vi "Attributes_DAQwfm.vi"(2 "data":waveform(dbl)[](array[waveform]), 3 "Refnum in":refnum<k21>) -> (0 "Array":waveform(dbl)[](array[waveform]), 1 "Refnum in 2":refnum<k21>)   [LabVIEW 2017]
uses:
  <resource>/objmgr/daqmx.rc
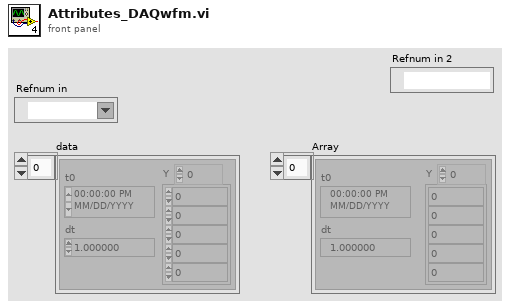
[diagram p1: front panel]
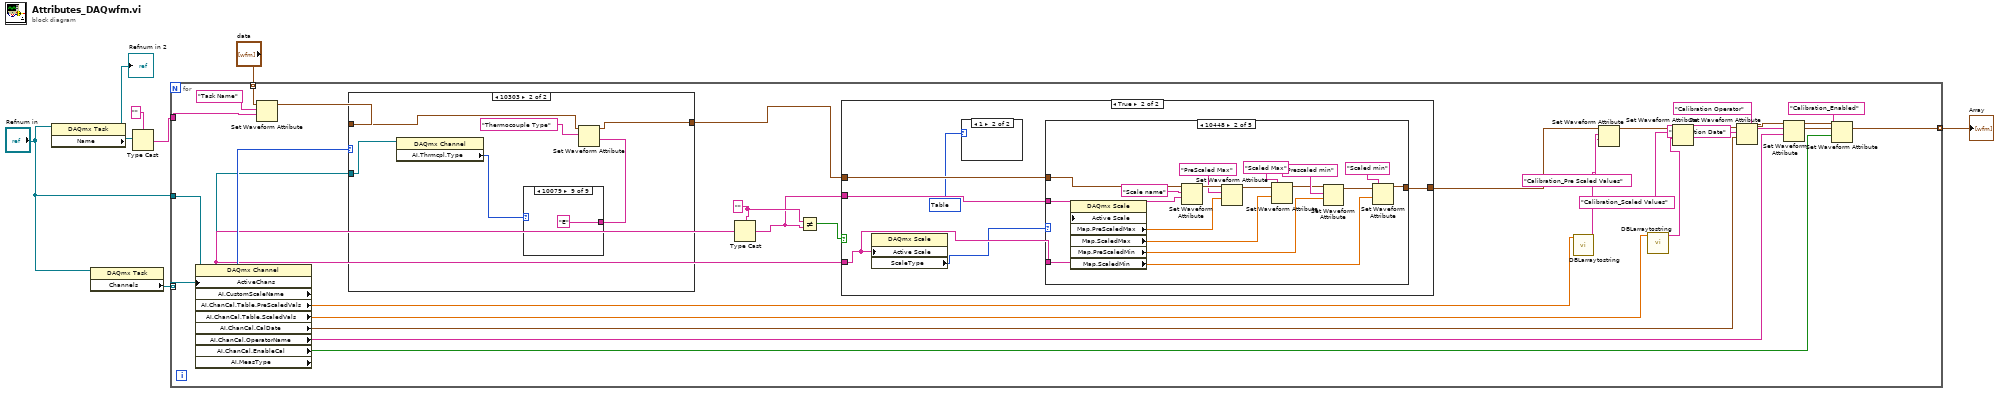
[diagram p0: block diagram]
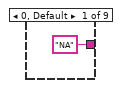
[diagram p3: hidden frame]
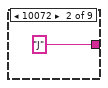
[diagram p4: hidden frame]
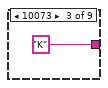
[diagram p5: hidden frame]
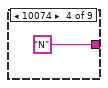
[diagram p6: hidden frame]
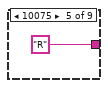
[diagram p7: hidden frame]
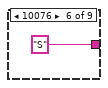
[diagram p8: hidden frame]
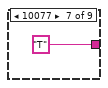
[diagram p9: hidden frame]
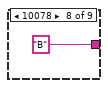
[diagram p10: hidden frame]
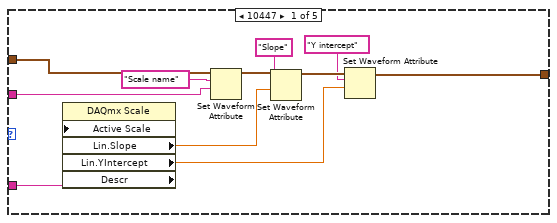
[diagram p13: hidden frame]
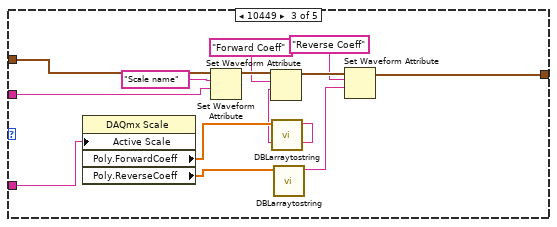
[diagram p14: hidden frame]
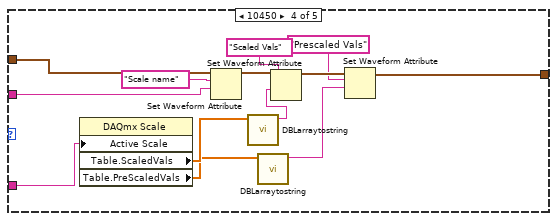
[diagram p15: hidden frame]
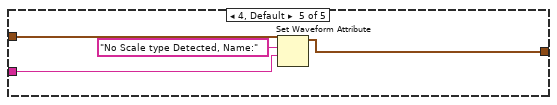
[diagram p16: hidden frame]
diagram:
  n1 = property class="DAQmx Task"(reference="Refnum in") -> (reference out=→"Refnum in 2":refnum<k21>, "Name"=w5:refnum<k21>)  [unwired: 1 in, 1 out]
  n2 = property class="DAQmx Task"(reference="Refnum in") -> ("Channels"=w2:refnum<k21>[])  [unwired: 1 in, 2 out]
  n3 = Type Cast(type="", x=w5) -> (*(type *) &x=w7:string)
  n4 = for {
    tunnel: "data" -> [w38] mode=indexing
    tunnel: [w19] -> w8 mode=indexing
    tunnel: w7 -> [w37]
    tunnel: "Refnum in" -> [w36]
    tunnel: w2 -> [w35] mode=indexing
    w18 = "" ("type")
    n5 = property class="DAQmx Channel"(reference=w36, "ActiveChans"=w35) -> (reference out=w12:refnum<k21>, "AI.CustomScaleName"=w13:tag, "AI.ChanCal.Table.PreScaledVals"=w30:dbl[], "AI.ChanCal.Table.ScaledVals"=w9:dbl[], "AI.ChanCal.CalDate"=w27:timestamp, "AI.ChanCal.OperatorName"=w25:string, "AI.ChanCal.EnableCal"=w23:bool, "AI.MeasType"=w14:i32)  [unwired: 1 in, 1 out]
    n6 = Set Waveform Attribute(5:w37, 6:"Task Name" ("name"), 7:w38) -> (3:w11:waveform(dbl))  [unwired: 1 in, 2 out]
    n7 = case shown="10303" w14 {
      tunnel: w12 -> [_ w46]
      tunnel: w11 -> [w40 w44]
      tunnel: [w40 w43] -> w10
      frame 0, Default {
      }
      frame 10303 {
        n8 = property class="DAQmx Channel"(reference=w46) -> ("AI.Thrmcpl.Type"=w42:i32)  [unwired: 1 in, 2 out]
        n9 = case shown="10079" w42 {
          tunnel: ["NA" "J" "K" "N" "R" "S" "T" "B" "E"] -> w41
          frame 0, Default {
          }
          frame 10072 {
          }
          frame 10073 {
          }
          frame 10074 {
          }
          frame 10075 {
          }
          frame 10076 {
          }
          frame 10077 {
          }
          frame 10078 {
          }
          frame 10079 {
          }
        }
        n10 = Set Waveform Attribute(5:w41, 6:"Thermocouple Type" ("name"), 7:w44) -> (3:w43:waveform(dbl))  [unwired: 1 in, 2 out]
      }
    }
    n11 = Type Cast(type=w18, x=w13) -> (*(type *) &x=w16:string)
    n12 = Not Equal?(x=w18, y=w16) -> (x != y?=w17:bool)
    n13 = case shown="True" w17 {
      tunnel: w10 -> [w56 w62]
      tunnel: [w56 w61] -> w31
      tunnel: w13 -> [_ w60]
      tunnel: w16 -> [_ w59]
      frame False {
      }
      frame True {
        w58 = 10450 items=["Linear"=10447, "Map Ranges"=10448, "Polynomial"=10449, "Table"=10450] ("ScaleType")
        n14 = property class="DAQmx Scale"("Active Scale"=w60) -> ("ScaleType"=w57:i32)  [unwired: 2 in, 2 out]
        n15 = case shown="1" w58 {
          frame 0, Default {
          }
          frame 1 {
          }
        }
        n16 = case shown="10448" w57 {
          tunnel: w62 -> [w73 w90 w103 w116 w120]
          tunnel: [w72 w76 w102 w115 w119] -> w61
          tunnel: w60 -> [w64 w82 w96 w109 _]
          tunnel: w59 -> [w63 w81 w95 w108 w117]
          frame 10447 {
            n17 = property class="DAQmx Scale" props=["Active Scale", "Lin.Slope", "Lin.YIntercept", "Descr"]("Active Scale"=w64) -> ("Lin.Slope"=w68:dbl, "Lin.YIntercept"=w67:dbl)  [unwired: 2 in, 3 out]
            n18 = Set Waveform Attribute(5:w63, 6:"Scale name" ("name"), 7:w73) -> (3:w70:waveform(dbl))  [unwired: 1 in, 2 out]
            n19 = Set Waveform Attribute(5:w68, 6:"Slope" ("name"), 7:w70) -> (3:w69:waveform(dbl))  [unwired: 1 in, 2 out]
            n20 = Set Waveform Attribute(5:w67, 6:"Y intercept" ("name"), 7:w69) -> (3:w72:waveform(dbl))  [unwired: 1 in, 2 out]
          }
          frame 10448 {
            n21 = property class="DAQmx Scale"("Active Scale"=w82) -> ("Map.PreScaledMax"=w86:dbl, "Map.ScaledMax"=w85:dbl, "Map.PreScaledMin"=w75:dbl, "Map.ScaledMin"=w74:dbl)  [unwired: 2 in, 2 out]
            n22 = Set Waveform Attribute(5:w81, 6:"Scale name" ("name"), 7:w90) -> (3:w88:waveform(dbl))  [unwired: 1 in, 2 out]
            n23 = Set Waveform Attribute(5:w86, 6:"PreScaled Max" ("name"), 7:w88) -> (3:w87:waveform(dbl))  [unwired: 1 in, 2 out]
            n24 = Set Waveform Attribute(5:w85, 6:"Scaled Max" ("name"), 7:w87) -> (3:w77:waveform(dbl))  [unwired: 1 in, 2 out]
            n25 = Set Waveform Attribute(5:w75, 6:"Prescaled min" ("name"), 7:w77) -> (3:w78:waveform(dbl))  [unwired: 1 in, 2 out]
            n26 = Set Waveform Attribute(5:w74, 6:"Scaled min" ("name"), 7:w78) -> (3:w76:waveform(dbl))  [unwired: 1 in, 2 out]
          }
          frame 10449 {
            n27 = property class="DAQmx Scale"("Active Scale"=w96) -> ("Poly.ForwardCoeff"=w94:dbl[], "Poly.ReverseCoeff"=w92:dbl[])  [unwired: 2 in, 2 out]
            n28 = Set Waveform Attribute(5:w95, 6:"Scale name" ("name"), 7:w103) -> (3:w100:waveform(dbl))  [unwired: 1 in, 2 out]
            n29 = call "DBLarraytostring.vi"("AI.ChanCal.Table.PreScaledVals"=w94) -> ("String"=w93:string)  [unwired: 10 in]
            n30 = Set Waveform Attribute(5:w93, 6:"Forward Coeff" ("name"), 7:w100) -> (3:w99:waveform(dbl))  [unwired: 1 in, 2 out]
            n31 = call "DBLarraytostring.vi"("AI.ChanCal.Table.PreScaledVals"=w92) -> ("String"=w91:string)  [unwired: 10 in]
            n32 = Set Waveform Attribute(5:w91, 6:"Reverse Coeff" ("name"), 7:w99) -> (3:w102:waveform(dbl))  [unwired: 1 in, 2 out]
          }
          frame 10450 {
            n33 = property class="DAQmx Scale"("Active Scale"=w109) -> ("Table.ScaledVals"=w107:dbl[], "Table.PreScaledVals"=w105:dbl[])  [unwired: 2 in, 2 out]
            n34 = Set Waveform Attribute(5:w108, 6:"Scale name" ("name"), 7:w116) -> (3:w113:waveform(dbl))  [unwired: 1 in, 2 out]
            n35 = call "DBLarraytostring.vi"("AI.ChanCal.Table.PreScaledVals"=w107) -> ("String"=w106:string)  [unwired: 10 in]
            n36 = call "DBLarraytostring.vi"("AI.ChanCal.Table.PreScaledVals"=w105) -> ("String"=w104:string)  [unwired: 10 in]
            n37 = Set Waveform Attribute(5:w106, 6:"Scaled Vals" ("name"), 7:w113) -> (3:w112:waveform(dbl))  [unwired: 1 in, 2 out]
            n38 = Set Waveform Attribute(5:w104, 6:"Prescaled Vals" ("name"), 7:w112) -> (3:w115:waveform(dbl))  [unwired: 1 in, 2 out]
          }
          frame 4, Default {
            n39 = Set Waveform Attribute(5:w117, 6:"No Scale type Detected, Name:" ("name"), 7:w120) -> (3:w119:waveform(dbl))  [unwired: 1 in, 2 out]
          }
        }
      }
    }
    n40 = call "DBLarraytostring.vi"("AI.ChanCal.Table.PreScaledVals"=w30) -> ("String"=w29:string)  [unwired: 10 in]
    n41 = Set Waveform Attribute(5:w29, 6:"Calibration_Pre Scaled Values" ("name"), 7:w31) -> (3:w34:waveform(dbl))  [unwired: 1 in, 2 out]
    n42 = call "DBLarraytostring.vi"("AI.ChanCal.Table.PreScaledVals"=w9) -> ("String"=w15:string)  [unwired: 10 in]
    n43 = Set Waveform Attribute(5:w15, 6:"Calibration_Scaled Values" ("name"), 7:w34) -> (3:w28:waveform(dbl))  [unwired: 1 in, 2 out]
    n44 = Set Waveform Attribute(5:w27, 6:"Calibration Date" ("name"), 7:w28) -> (3:w21:waveform(dbl))  [unwired: 1 in, 2 out]
    n45 = Set Waveform Attribute(5:w25, 6:"Calibration Operator" ("name"), 7:w21) -> (3:w20:waveform(dbl))  [unwired: 1 in, 2 out]
    n46 = Set Waveform Attribute(5:w23, 6:"Calibration_Enabled" ("name"), 7:w20) -> (3:w19:waveform(dbl))  [unwired: 1 in, 2 out]
  }
  "Array" <- w8
